vi "extract_singal_channel_data.vi"(8 "data in":waveform(dbl)[](array[waveform]), 9 "Array - Numeric":dbl[](array[numeric]), 10 "?":T1(array[cluster]) {"Terminal Configuration" items=["default"=-1, "RSE"=10083, "NRSE"=10078, "Differential"=10106, "Pseudodifferential"=12529]}, 11 "channel index":dbl) -> (2 "data out":waveform(dbl)[](array[waveform]))   [LabVIEW 2024]
panel:
  in  "element":waveform(dbl)
  in  "vaild channel":dbl
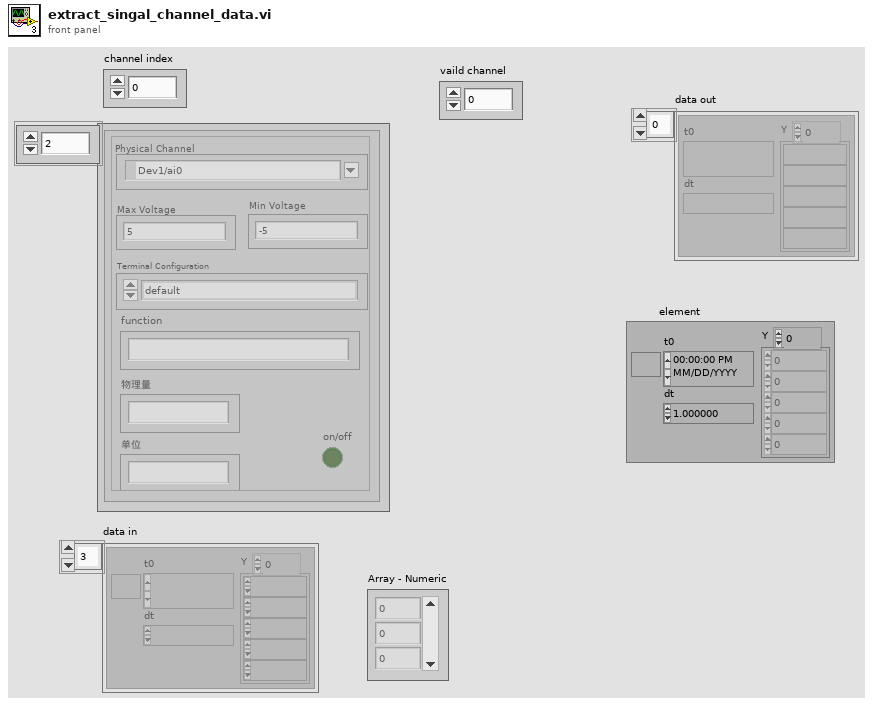
[diagram p1: front panel]
types:
  T1 = cluster{"Terminal Configuration":i32, "Min Voltage":dbl, "Physical Channel":tag, "Max Voltage":dbl, "function":string, "on/off":bool, "物理量":string, "单位":string}[]
  T2 = cluster{"Terminal Configuration":i32, "Min Voltage":dbl, "Physical Channel":tag, "Max Voltage":dbl, "function":string, "on/off":bool, "物理量":string, "单位":string}
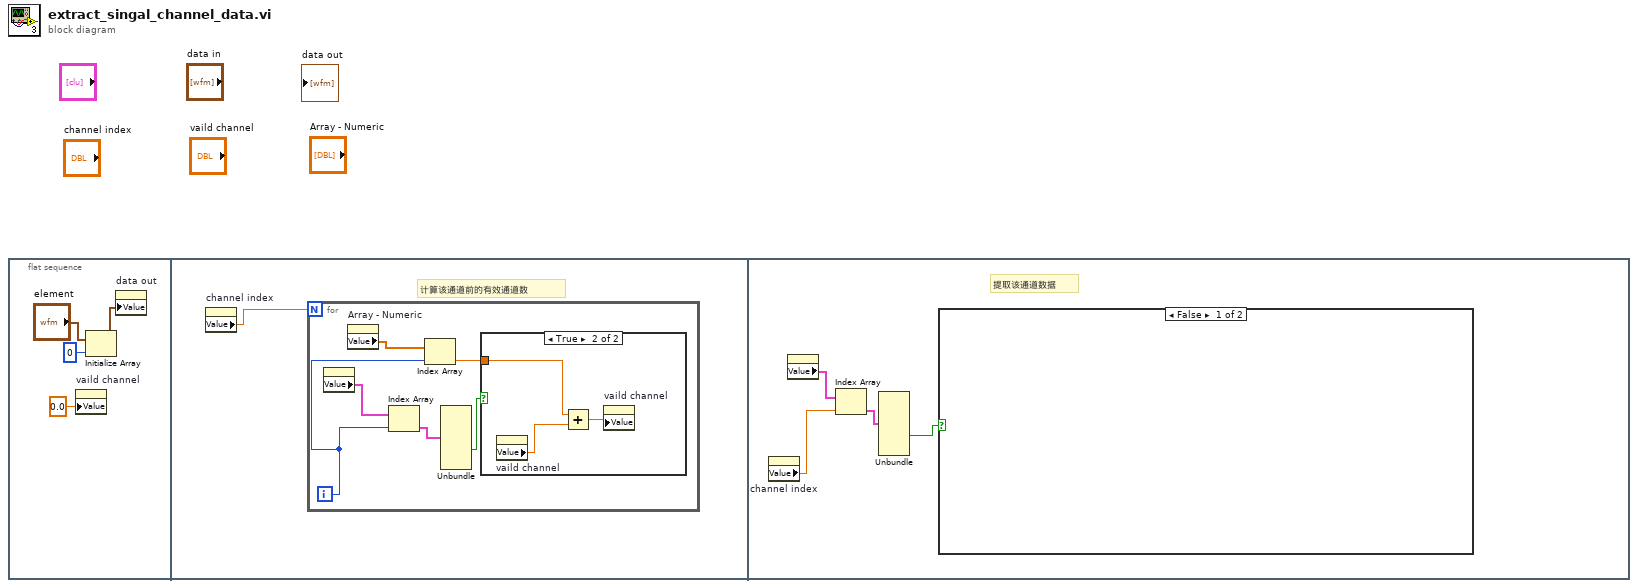
[diagram p0: block diagram]
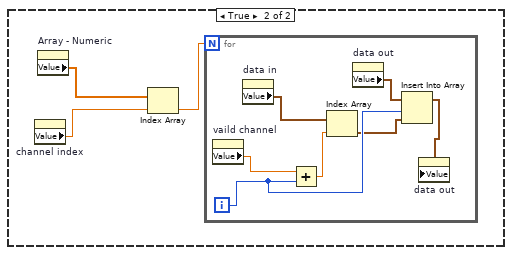
[diagram p3: hidden frame]
diagram:
  n1 = flat-sequence {
    frame #0 {
      n2 = property on="vaild channel" class="DigNum (strict)"("Value"=0.0 ("vaild channel")) -> ()  [unwired: 2 in, 2 out]
      n3 = Initialize Array("element", 0 ("dimension size")) -> (w1:waveform(dbl)[])
      n4 = property on="data out" class="Arr (strict)"("Value"=w1) -> ()  [unwired: 2 in, 2 out]
    }
    frame #1 {
      # "计算该通道前的有效通道数"
      n5 = property on="channel index" class="DigNum (strict)"() -> ("Value"=w5:dbl)  [unwired: 2 in, 2 out]
      n6 = for {
        N: w5 -> [_]
        i -> [w8]
        n7 = property class="Arr (strict)"() -> ("Value"=w11:T1)  [unwired: 2 in, 2 out]
        n8 = property on="Array - Numeric" class="Arr (strict)"() -> ("Value"=w9:dbl[])  [unwired: 2 in, 2 out]
        n9 = Index Array(array=w11, index=w8) -> (element=w10:T2)
        n10 = Index Array(array=w9, index=w8) -> (element=w6:dbl)
        n11 = Unbundle(w10) -> ("on/off"=w7:bool)  [unwired: 7 out]
        n12 = case shown="True" w7 {
          tunnel: w6 -> [_ w13]
          frame False {
          }
          frame True {
            n13 = property on="vaild channel" class="DigNum (strict)"() -> ("Value"=w14:dbl)  [unwired: 2 in, 2 out]
            n14 = Add(x=w13, y=w14) -> (x+y=w12:dbl)
            n15 = property on="vaild channel" class="DigNum (strict)"("Value"=w12) -> ()  [unwired: 2 in, 2 out]
          }
        }
      }
    }
    frame #2 {
      # "提取该通道数据"
      n16 = property on="channel index" class="DigNum (strict)"() -> ("Value"=w17:dbl)  [unwired: 2 in, 2 out]
      n17 = property class="Arr (strict)"() -> ("Value"=w18:T1)  [unwired: 2 in, 2 out]
      n18 = Index Array(array=w18, index=w17) -> (element=w16:T2)
      n19 = Unbundle(w16) -> ("on/off"=w15:bool)  [unwired: 7 out]
      n20 = case shown="False" w15 {
        frame False {
        }
        frame True {
          n21 = property on="channel index" class="DigNum (strict)"() -> ("Value"=w20:dbl)  [unwired: 2 in, 2 out]
          n22 = property on="Array - Numeric" class="Arr (strict)"() -> ("Value"=w21:dbl[])  [unwired: 2 in, 2 out]
          n23 = Index Array(array=w21, index=w20) -> (element=w19:dbl)
          n24 = for {
            N: w19 -> [_]
            i -> [w25]
            n25 = property on="vaild channel" class="DigNum (strict)"() -> ("Value"=w28:dbl)  [unwired: 2 in, 2 out]
            n26 = property on="data in" class="Arr (strict)"() -> ("Value"=w27:waveform(dbl)[])  [unwired: 2 in, 2 out]
            n27 = Add(x=w28, y=w25) -> (x+y=w26:dbl)
            n28 = Index Array(array=w27, index=w26) -> (element=w23:waveform(dbl))
            n29 = property on="data out" class="Arr (strict)"() -> ("Value"=w24:waveform(dbl)[])  [unwired: 2 in, 2 out]
            n30 = Insert Into Array(array=w24, index=w25, new element=w23) -> (w22:waveform(dbl)[])
            n31 = property on="data out" class="Arr (strict)"("Value"=w22) -> ()  [unwired: 2 in, 2 out]
          }
        }
      }
    }
  }
